vi "App - link RPR V2.vi"() -> ()   [LabVIEW 2014]
uses:
  link input file header.ctl
  link -- rusout.ctl
  <vilib>/Utility/file.llb/Write To Spreadsheet File (string).vi
panel:
  in  "RPR Cyl folder Path":path=path "C:/data/RUS/Experiment/ProbeTest/Probe10/YBCO_5/singlesweep/RPR"
  in  "Tab : calculate":T1(tab)=enum."calculate rusin"
  in  "calculate whatever":bool
  in  "READ rusout 2":string="rusout - U1 - 350K.dat"
  in  "READ rusout 1":string="rusout - U1 - 300K.dat"
  in  "# of peaks to use":i32=21
  out "delta log c11  opt":dbl
  out "delta log c44  opt":dbl
  out "size(s)":i32
  out "delta log c11  fit":dbl
  out "delta log c44  fit":dbl
  out "delta log bulk":dbl
  out "rusout out":T2
  out "bulk modulus":dbl
  in  "delta T":dbl
  out "d log c11  / dT":dbl
  out "d log c44  / dT 2":dbl
  out "d log B  / dT 2":dbl
  in  "executable":string="Cyl8.exe"
  out "Plot: measured":cluster{"all rows":dbl[], "all rows":dbl[]}[](graph)=[{"all rows"=[0.0, 0.0], "all rows"=[1.1, 2.0]}, {"all rows"=[0.56242053, 0.56242053], "all rows"=[1.1, 2.0]}, {"all rows"=[0.64670384, 0.64670384], "all rows"=[1.1, 2.0]}, {"all rows"=[0.9732775, 0.9732775], "all rows"=[1.1, 2.0]}, {"all rows"=[1.12840965, 1.12840965], "all rows"=[1.1, 2.0]}, {"all rows"=[1.20822828, 1.20822828], "all rows"=[1.1, 2.0]}, {"all rows"=[1.57768763, 1.57768763], "all rows"=[1.1, 2.0]}, {"all rows"=[1.57768763, 1.57768763], "all rows"=[1.1, 2.0]}, {"all rows"=[1.7632479699999999, 1.7632479699999999], "all rows"=[1.1, 2.0]}, {"all rows"=[1.8181119799999998, 1.8181119799999998], "all rows"=[1.1, 2.0]}, {"all rows"=[1.86633313, 1.86633313], "all rows"=[1.1, 2.0]}, {"all rows"=[1.89548067, 1.89548067], "all rows"=[1.1, 2.0]}, {"all rows"=[1.99767853, 1.99767853], "all rows"=[1.1, 2.0]}, {"all rows"=[2.13077551, 2.13077551], "all rows"=[1.1, 2.0]}, {"all rows"=[2.21863208, 2.21863208], "all rows"=[1.1, 2.0]}, {"all rows"=[2.25352052, 2.25352052], "all rows"=[1.1, 2.0]}, {"all rows"=[2.34897001, 2.34897001], "all rows"=[1.1, 2.0]}, {"all rows"=[2.44704923, 2.44704923], "all rows"=[1.1, 2.0]}, {"all rows"=[2.56952625, 2.56952625], "all rows"=[1.1, 2.0]}, {"all rows"=[2.80714819, 2.80714819], "all rows"=[1.1, 2.0]}, {"all rows"=[2.96152034, 2.96152034], "all rows"=[1.1, 2.0]}, {"all rows"=[3.11746088, 3.11746088], "all rows"=[1.1, 2.0]}, {"all rows"=[3.31568501, 3.31568501], "all rows"=[1.1, 2.0]}, {"all rows"=[3.4544333099999998, 3.4544333099999998], "all rows"=[1.1, 2.0]}]
  in  "Y Path":path=path "C:/data/RUS/Experiment/ProbeTest/Probe10/YBCO_5/singlesweep/RPR"
  in  "READ Y file":string="for_RPR.dat"
  in  "# of peaks to show":i32=21
  in  "Color Box":u32(colorbox)
  out "Plot: fitted":cluster{"all rows":dbl[], "all rows":dbl[]}[](graph)=[{"all rows"=[0.0, 0.0], "all rows"=[0.0, 1.0]}]
  in  "X Scale.Range:Maximum":dbl
  in  "READ rusout":string="rusout.dat"
  in  "WRITE rusin":string="rusin.dat"
  in  "calculate rusin":bool
  in  "rusin header":T3={"number of moduli"="6", "number of dimensions"="3", "order of the basic set"="14", "fit/calculate"="20", "mass (gram)"="0.0008", "convergence "="10", "output to"="1", "free to float"="0 0 0 0 0 0 0 0 0 ", "guesses"="2.31 2.68 1.86 0.95 0.71 1.00 0.39 0.37 0.95 ", "dimensions"="0.083  0.097  0.016", "comment line"="comment "}
  out "rusout exists?":bool=TRUE
  out "standard output":string
  out "standard error":string
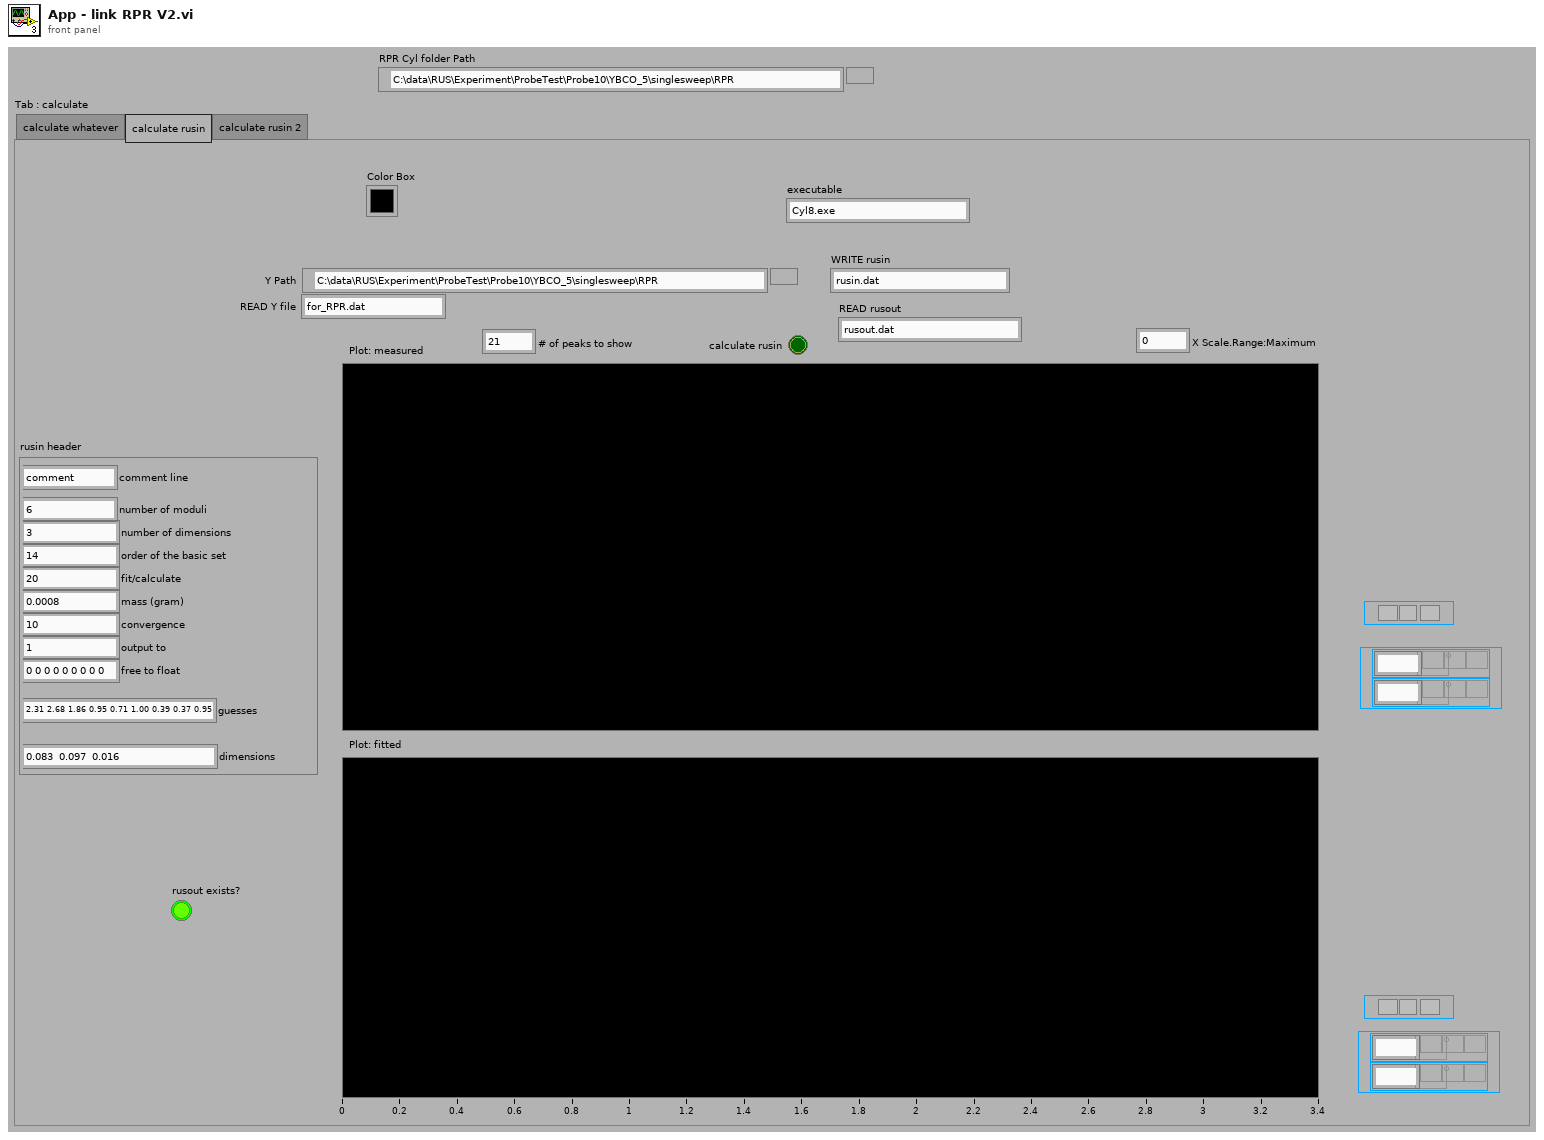
[diagram p1: front panel]
types:
  T1 = enum32{"calculate whatever", "calculate rusin", "calculate rusin 2"}
  T2 = typedef "link -- rusout.ctl" = cluster{"freqs Exp":dbl[], "symmetry":i32[], "dmod11":dbl[], "dmod44":dbl[], "freqs Fit":dbl[], "header":string, "bulk modulus":dbl, "c11":dbl, "c44":dbl}
  T3 = typedef "link input file header.ctl" = cluster{"number of moduli":string, "number of dimensions":string, "order of the basic set":string, "fit/calculate":string, "mass (gram)":string, "convergence ":string, "output to":string, "free to float":string, "guesses":string, "dimensions":string, "comment line":string}
  T4 = cluster{"Name":string, "Color":u32, "Style":u8, "Point Style":u8, "Name Visible":bool, "Allow Drag":bool, "Annotation Mode":u32, "Plot":i32, "Index":i32, "Position":cluster{"X":dbl, "Y":dbl}, "X Scale":u32, "Y Scale":u32, "Show Arrow":bool, "Lock Name":bool, "Plot Area":i32, "Label Offset":cluster{"X":dbl, "Y":dbl}}[]
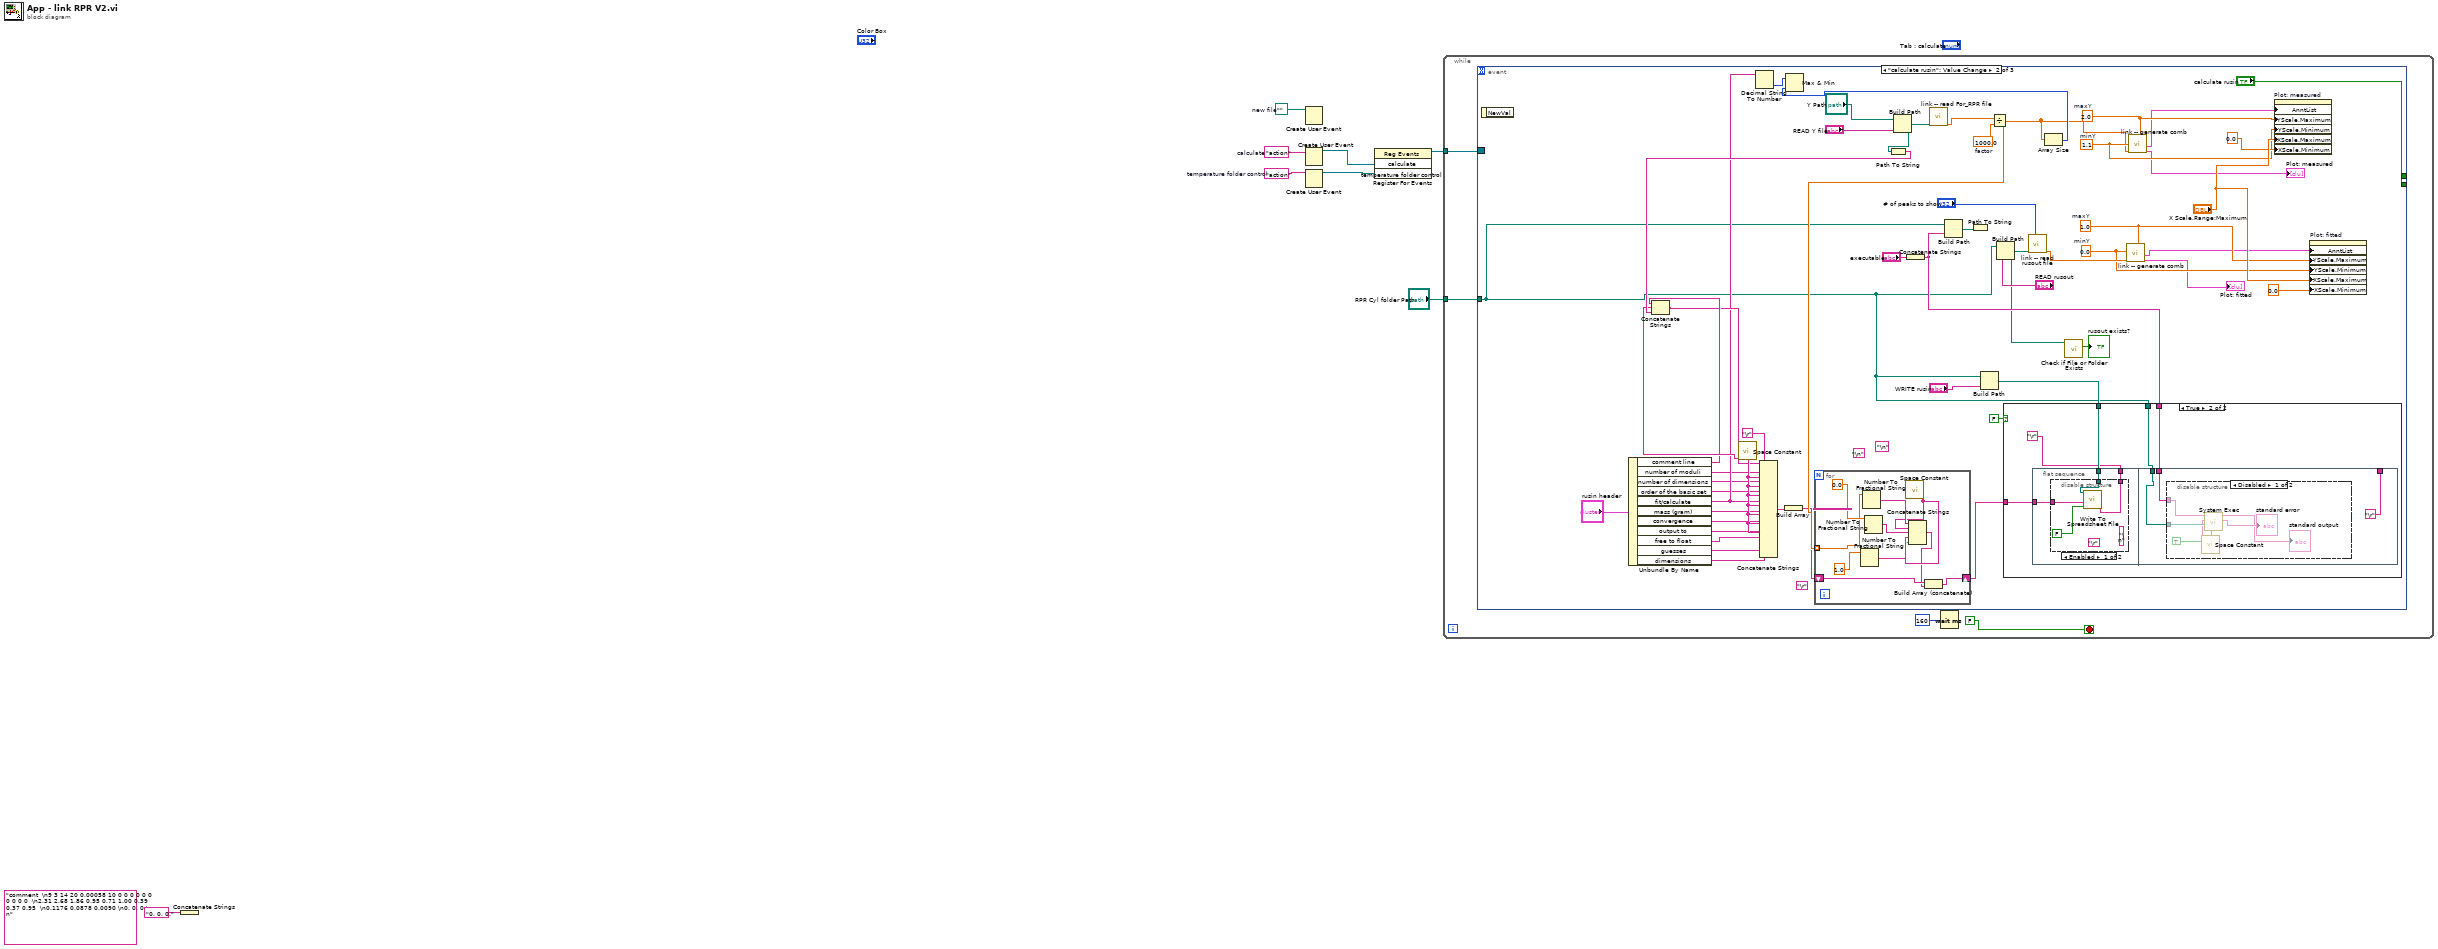
[diagram p0: block diagram]
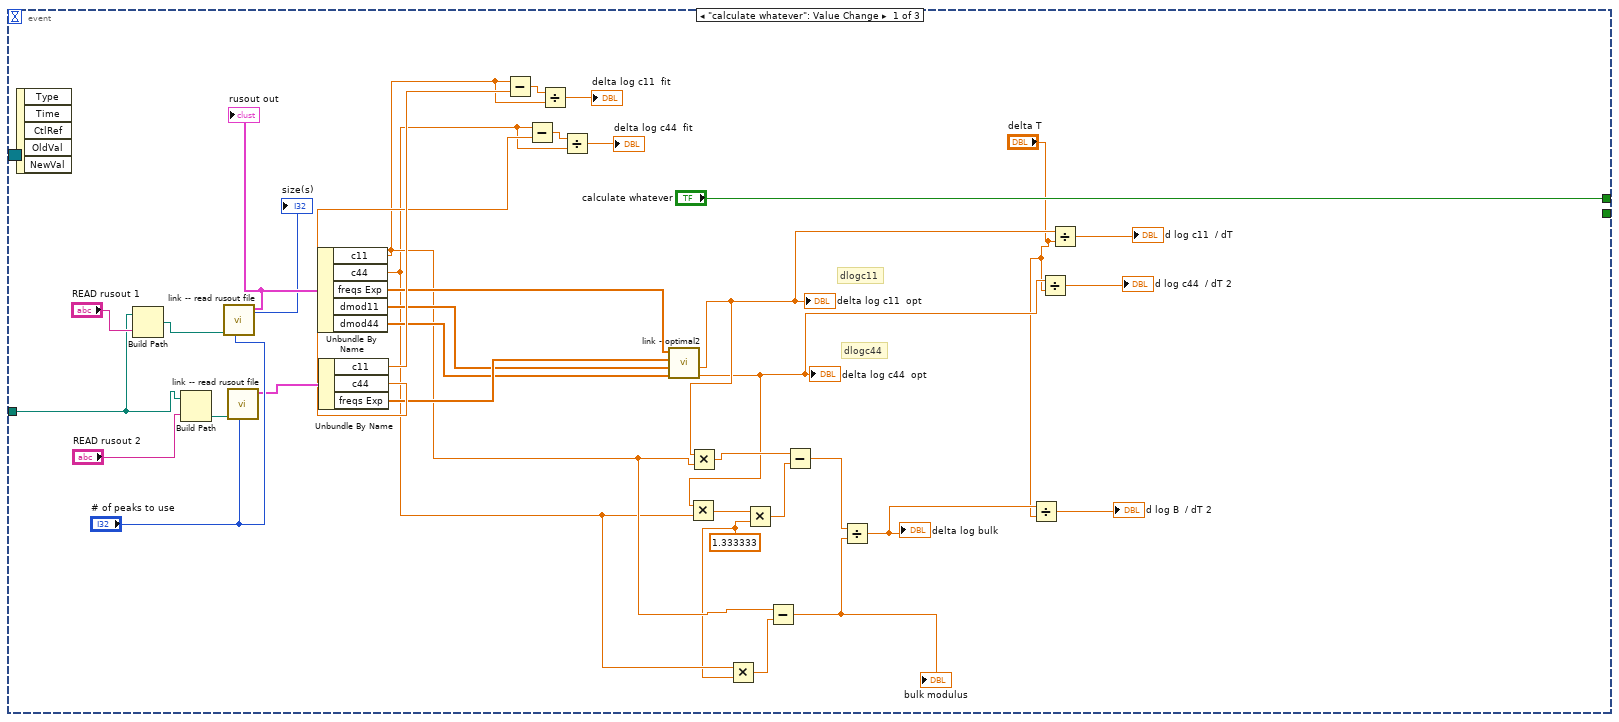
[diagram p2: hidden frame]
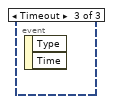
[diagram p6: hidden frame]
diagram:
  w3 = "action"  # calculate
  w5 = "action"  # temperature folder control
  w6 = path ""  # new file
  (unwired) "comment  \n9 3 14 20 0.00058 10 0 0 0 0 0 0 0 0 0 0  \n2.31 2.68 1.86 0.95 0.71 1.00 0.39 0.37 0.95  \n0.1176 0.0878 0.0090 \n0. 0. 0.\n" ("string")
  n1 = Concatenate Strings("0. 0. 0." ("string")) -> ()  [unwired: 1 out]
  n2 = Create User Event(user event datatype=w6) -> ()  [unwired: 1 in, 2 out]
  n3 = Create User Event(user event datatype=w3) -> (user event=w7:refnum<user-event>)  [unwired: 1 in, 1 out]
  n4 = Create User Event(user event datatype=w5) -> (user event=w4:refnum<user-event>)  [unwired: 1 in, 1 out]
  n5 = register-events(w7, w4) -> (reference out=w2:refnum<event-registration>)  [unwired: 2 in, 1 out]
  n6 = while {
    tunnel: w2 -> [w12]
    tunnel: "RPR Cyl folder Path" -> [w9]
    stop <- FALSE stop-if-true
    n7 = event shown="[1] \"calculate rusin\": Value Change" {
      selector: w12 -> [_ _ _]
      dyn-events: _ -> [_ _ _]
      timeout: _ -> [_ _ _]
      tunnel: ["calculate whatever" _ _] -> _
      tunnel: w9 -> [w44 w53 _]
      tunnel: [_ "calculate rusin" _] -> _
      event "calculate whatever": Value Change {
        w22 = 1.333333
        # "dlogc44"
        # "dlogc11"
        n8 = event-data() -> ()  [unwired: 1 in, 5 out]
        n9 = Build Path(base path=w44, name or relative path="READ rusout 1") -> (appended path=w43:path)
        n10 = Build Path(base path=w44, name or relative path="READ rusout 2") -> (appended path=w47:path)
        n11 = call "link -- read rusout file.vi"("# of peaks to show"="# of peaks to use", "rus out file path"=w43) -> ("rusout out"=w41:T2, "size(s)"=→"size(s)":i32)  [unwired: 7 in, 1 out]
        "rusout out" <- w41
        n12 = call "link -- read rusout file.vi"("# of peaks to show"="# of peaks to use", "rus out file path"=w47) -> ("rusout out"=w40:T2)  [unwired: 7 in, 2 out]
        n13 = Unbundle By Name(w41) -> ("c11"=w24:dbl, "c44"=w23:dbl, "freqs Exp"=w31:dbl[], "dmod11"=w30:dbl[], "dmod44"=w29:dbl[])
        n14 = Unbundle By Name(w40) -> ("c11"=w37:dbl, "c44"=w33:dbl, "freqs Exp"=w32:dbl[])
        n15 = Subtract(x=w24, y=w37) -> (x-y=w38:dbl)
        n16 = Subtract(x=w23, y=w33) -> (x-y=w35:dbl)
        n17 = Divide(x=w38, y=w24) -> (x/y=→"delta log c11  fit":dbl)
        n18 = Divide(x=w35, y=w23) -> (x/y=→"delta log c44  fit":dbl)
        n19 = call "link - optimal2.vi"("dc44"=w29, "dc11"=w30, "freqs 2"=w32, "freqs 1"=w31) -> ("beta opt"=w16:dbl, "alpha opt"=w19:dbl)  [unwired: 6 in]
        "delta log c11  opt" <- w19
        "delta log c44  opt" <- w16
        n20 = Multiply(x=w16, y=w23) -> (x*y=w27:dbl)
        n21 = Multiply(x=w19, y=w24) -> (x*y=w28:dbl)
        n22 = Multiply(x=w23, y=w22) -> (x*y=w25:dbl)
        n23 = Multiply(x=w27, y=w22) -> (x*y=w26:dbl)
        n24 = Subtract(x=w24, y=w25) -> (x-y=w20:dbl)
        "bulk modulus" <- w20
        n25 = Subtract(x=w28, y=w26) -> (x-y=w21:dbl)
        n26 = Divide(x=w21, y=w20) -> (x/y=w14:dbl)
        "delta log bulk" <- w14
        n27 = Divide(x=w14, y="delta T") -> (x/y=→"d log B  / dT 2":dbl)
        n28 = Divide(x=w16, y="delta T") -> (x/y=→"d log c44  / dT 2":dbl)
        n29 = Divide(x=w19, y="delta T") -> (x/y=→"d log c11  / dT":dbl)
      }
      event "calculate rusin": Value Change {
        w74 = 1000.0  # factor
        w83 = 2.0  # maxY
        w84 = 1.1  # minY
        w86 = 1.0  # maxY
        w87 = 0.0  # minY
        (unwired) "\n"
        (unwired) "\n"
        (unwired) "\r"
        w52 = "\r"
        n30 = event-data() -> ()  [unwired: 1 in, 1 out]
        n31 = Unbundle By Name("rusin header") -> ("comment line"=w92:string, "number of moduli"=w57:string, "number of dimensions"=w58:string, "order of the basic set"=w59:string, "fit/calculate"=w71:string, "mass (gram)"=w60:string, "convergence"=w61:string, "output to"=w62:string, "free to float"=w63:string, "guesses"=w64:string, "dimensions"=w65:string)
        n32 = call <vilib>:"Space Constant.vi"() -> ("String"=w93:string)
        n33 = Decimal String To Number(string=w71) -> (number=w78:i32)  [unwired: 2 in, 1 out]
        n34 = Build Path(base path="Y Path", name or relative path="READ Y file") -> (appended path=w96:path)
        n35 = Path To String(path=w96) -> (string=w94:string)
        n36 = Concatenate Strings(w92, w93, w94) -> (w91:string)
        n37 = Concatenate Strings(w91, w52, w57, w93, w58, w93, w59, w93, w71, w93, w60, w93, w61, w93, w62, w93, w63, w52, w64, w52, w65) -> (w69:string)
        n38 = Build Array(w69) -> (w75:string[])
        n39 = Concatenate Strings("executable") -> (w68:string)
        n40 = call "link -- read For_RPR file.vi"("rus out file path"=w96) -> ("freqs"=w95:dbl[])  [unwired: 10 in]
        n41 = Build Path(base path=w53, name or relative path=w68) -> (appended path=w55:path)
        n42 = Path To String(path=w55) -> ()  [unwired: 1 out]
        n43 = Build Path(base path=w53, name or relative path="WRITE rusin") -> (appended path=w67:path)
        n44 = Divide(x=w95, y=w74) -> (x/y=w77:dbl[])
        n45 = for {
          tunnel: w77 -> [w121] mode=indexing
          shift-right: [w123] -> w76
          shift-left: w75 -> [w125]
          n46 = Number To Fractional String(number=1.0) -> (F-format string=w126:string)  [unwired: 3 in]
          n47 = Number To Fractional String(number=w121) -> (F-format string=w129:string)  [unwired: 3 in]
          n48 = Number To Fractional String(number=0.0) -> (F-format string=w128:string)  [unwired: 3 in]
          n49 = call <vilib>:"Space Constant.vi"() -> ("String"=w127:string)
          n50 = Concatenate Strings(w129, w127, w128, w127, w126) -> (w124:string)
          n51 = Build Array (concatenate)(w125, w124) -> (w123:string[])
        }
        n52 = Build Path(base path=w53, name or relative path="READ rusout") -> (appended path=w50:path)
        n53 = case shown="True" FALSE {
          tunnel: w76 -> [_ w104]
          tunnel: w68 -> [_ w103]
          tunnel: w67 -> [_ w102]
          tunnel: w53 -> [_ w101]
          frame False {
          }
          frame True {
            n54 = flat-sequence {
              tunnel: w104 -> [w107]
              tunnel: w102 -> [w106]
              tunnel: "\r" -> [w105]
              tunnel: w101 -> [w114]
              tunnel: w103 -> [w113]
              tunnel: ["\r"] -> _
              frame #0 {
                n55 = disable-structure shown="Enabled" {
                  disable-tunnel: w107 -> [w110 _]
                  disable-tunnel: w106 -> [w109 _]
                  disable-tunnel: w105 -> [w108 _]
                  frame Enabled {
                    (unwired) "\n" ("string")
                    (unwired) "\r"
                    n56 = call-poly <vilib>:"Write To Spreadsheet File.vi"("delimiter (\\t)"=w108, "append to file? (new file:F)"=FALSE, "1D data"=w110, "file path (dialog if empty)"=w109) -> ()  [unwired: 4 in, 1 out]
                  }
                  frame Disabled {
                  }
                }
              }
              frame #1 {
                n57 = disable-structure shown="Disabled" {
                  disable-tunnel: w114 -> [w120 _]
                  disable-tunnel: w113 -> [w119 _]
                  frame Disabled {
                    w118 = TRUE ("wait until completion? (T)")
                    n58 = call <vilib>:"Space Constant.vi"() -> ("String"=w117:string)
                    n59 = call <vilib>:"System Exec.vi"("run minimized? (F)"=w118, "wait until completion? (T)"=w118, "working directory"=w120, "standard input"=w117, "command line"=w119) -> ("standard error"=→"standard error":string, "standard output"=→"standard output":string)  [unwired: 3 in, 2 out]
                  }
                  frame Enabled {
                  }
                }
              }
            }
          }
        }
        n60 = call "link -- read rusout file.vi"("# of peaks to show"="# of peaks to show", "rus out file path"=w50) -> ("freqs"=w97:dbl[])  [unwired: 7 in, 2 out]
        n61 = Array Size(array=w77) -> (size(s)=w79:i32)
        n62 = Max & Min(x=w78, y=w79) -> ()  [unwired: 2 out]
        n63 = call <vilib>:"Check if File or Folder Exists.vi"("path"=w50) -> ("file or folder exists?"=→"rusout exists?":bool)  [unwired: 8 in, 2 out]
        n64 = call "link -- generate comb.vi"("maxY"=w86, "minY"=w87, "freq array"=w97) -> ("plot list"=→"Plot: fitted":cluster{dbl[], dbl[]}[], "annotation list"=w85:T4)  [unwired: 7 in]
        n65 = call "link -- generate comb.vi"("maxY"=w83, "minY"=w84, "freq array"=w77) -> ("plot list"=→"Plot: measured":cluster{dbl[], dbl[]}[], "annotation list"=w82:T4)  [unwired: 7 in]
        n66 = property on="Plot: measured" class="XYGraph (strict)"("AnntList"=w82, "YScale.Maximum"=w83, "YScale.Minimum"=w84, "XScale.Maximum"="X Scale.Range:Maximum", "XScale.Minimum"=0.0 ("X Scale.Range:Maximum")) -> ()  [unwired: 2 in, 2 out]
        n67 = property on="Plot: fitted" class="XYGraph (strict)"("AnntList"=w85, "YScale.Maximum"=w86, "YScale.Minimum"=w87, "XScale.Maximum"="X Scale.Range:Maximum", "XScale.Minimum"=0.0 ("X Scale.Range:Maximum")) -> ()  [unwired: 2 in, 2 out]
      }
      event Timeout {
        n68 = event-data() -> ()  [unwired: 1 in, 2 out]
      }
    }
    n69 = Wait (ms)(milliseconds to wait=u32 160) -> ()  [unwired: 1 out]
  }
